vi "Write Coil.vi"(8 "error in (no error)":errorcluster, 10 "Boolean":bool, 11 "DAM0404D in":refnum<class "DAM0404D.lvclass">) -> (0 "error out":errorcluster, 3 "DAM0404D out":refnum<class "DAM0404D.lvclass">)   [LabVIEW 2016, in "DAM0404D.lvlib" / "DAM0404D.lvclass"]
uses:
  DAM0404D.lvclass
  DAM0404D.lvclass/DAM0404D.ctl
  <vilib>/Plasmionique/MB Master/MB Master.lvlib
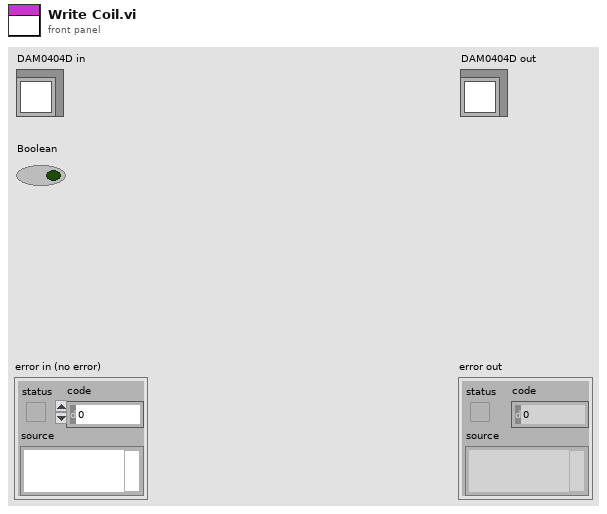
[diagram p1: front panel]
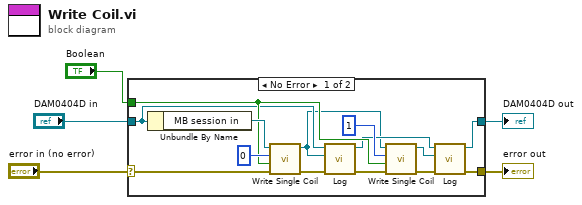
[diagram p0: block diagram]
diagram:
  n1 = case shown="No Error" "error in (no error)" {
    selector: "error in (no error)" -> [w18 w21]
    tunnel: [w8 w21] -> w4
    tunnel: [w9 w20] -> w2
    tunnel: "DAM0404D in" -> [w12 w20]
    tunnel: "Boolean" -> [w15 _]
    frame No Error {
      n2 = Unbundle By Name(w12) -> ("MB session in"=w19:refnum<class "MB_Master.lvclass">)
      n3 = call <vilib>:"Write Single Coil.vi"("error in (no error)"=w18, "value"=w15, "address"=u16 0, "MB session in"=w19) -> ("error out"=w14:errorcluster, "MB session out"=w7:refnum<class "MB_Master.lvclass">)  [unwired: 6 in]
      n4 = call "Log.vi"("error in (no error)"=w14, "MB session in"=w7, "DAM0404D in"=w12) -> ("error out"=w13:errorcluster, "DAM0404D out"=w10:refnum<class "DAM0404D.lvclass">)  [unwired: 7 in]
      n5 = call <vilib>:"Write Single Coil.vi"("error in (no error)"=w13, "value"=w15, "address"=u16 1, "MB session in"=w7) -> ("error out"=w11:errorcluster, "MB session out"=w6:refnum<class "MB_Master.lvclass">)  [unwired: 6 in]
      n6 = call "Log.vi"("error in (no error)"=w11, "MB session in"=w6, "DAM0404D in"=w10) -> ("error out"=w8:errorcluster, "DAM0404D out"=w9:refnum<class "DAM0404D.lvclass">)  [unwired: 7 in]
    }
    frame Error {
    }
  }
  "error out" <- w4
  "DAM0404D out" <- w2
